vi "DQMH-GenNet Dequeue Message.vi"(8 "error in":errorcluster, 11 "Message Queue in":refnum<class "DQMH-GenNet Message Queue.lvclass">) -> (0 "error out":errorcluster, 1 "Message Data":variant, 2 "Message":string, 3 "Message Queue out":refnum<class "DQMH-GenNet Message Queue.lvclass">)   [LabVIEW 2022 SP3, in "hse-gennet.lvlib" / "DQMH-GenNet Message Queue.lvclass"]
doc: "This VI pulls messages off the DQMH Generic Networking Message Queue.\n\n____\nHAMPEL SOFTWARE ENGINEERING v3.8.0 (2023-12-18 14:41)"
uses:
  DQMH-GenNet Message Queue.lvclass
  DQMH-GenNet Message Queue.lvclass/DQMH-GenNet Message Queue.ctl
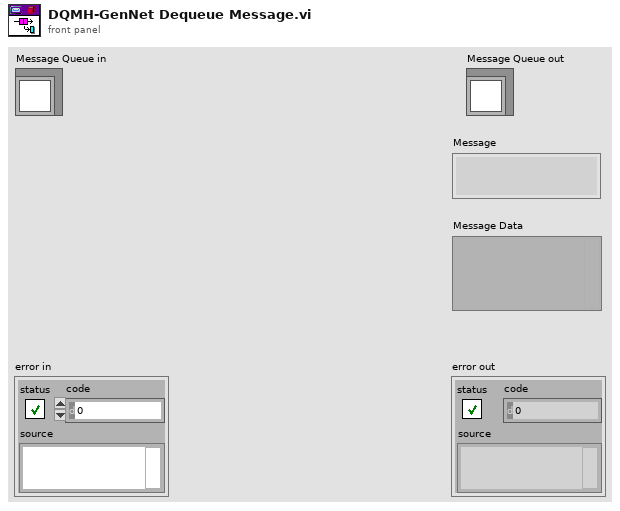
[diagram p1: front panel]
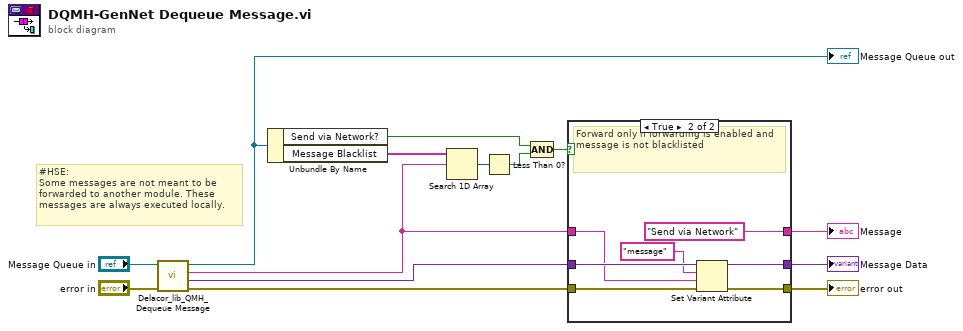
[diagram p0: block diagram]
diagram:
  # "#HSE: \nSome messages are not meant to be\nforwarded to another module. These\nmessages are always executed locally."
  n1 = call-dynamic "Delacor_lib_QMH_Dequeue Message.vi"("error in"="error in", "Message Queue in"="Message Queue in") -> ("error out"=w8:errorcluster, "Message Data"=w10:variant, "Message"=w6:string, "Message Queue out"=w12:refnum<class "DQMH-GenNet Message Queue.lvclass">)  [unwired: 6 in]
  "Message Queue out" <- w12
  n2 = Unbundle By Name(w12) -> ("Send via Network?"=w5:bool, "Message Blacklist"=w1:string[])
  n3 = Search 1D Array(1D array=w1, element=w6) -> (index of element=w3:i32)  [unwired: 1 in]
  n4 = Less Than 0?(x=w3) -> (x < 0?=w2:bool)
  n5 = Compound Arithmetic op=AND(w5, w2) -> (w4:bool)
  n6 = case shown="True" w4 {
    tunnel: [w16 "Send via Network" ("Message")] -> w11
    tunnel: [w17 w22] -> w9
    tunnel: w10 -> [w17 w23]
    tunnel: w6 -> [w16 w20]
    tunnel: w8 -> [w15 w19]
    tunnel: [w15 w18] -> w7
    frame False {
      # "forwarding disabled or message in blacklist"
    }
    frame True {
      # "Forward only if forwarding is enabled and message is not blacklisted"
      n7 = Set Variant Attribute(Variant=w23, name="message", value=w20, error in=w19) -> (Variant out=w22:variant, error out=w18:errorcluster)  [unwired: 1 out]
    }
  }
  "error out" <- w7
  "Message" <- w11
  "Message Data" <- w9
